vi "WebPowerSwitch.vi"() -> ()   [LabVIEW 2016]
uses:
  <vilib>/httpClient/LabVIEWHTTPClient.lvlib
panel:
  in  "url 2":string="http://LV:LV@192.168.126.155/outlet?a=OFF"
  out "error out":errorcluster
  out "body":string
  out "headers":string
  in  "url":string="http://LV:LV@192.168.126.155/index.htm"
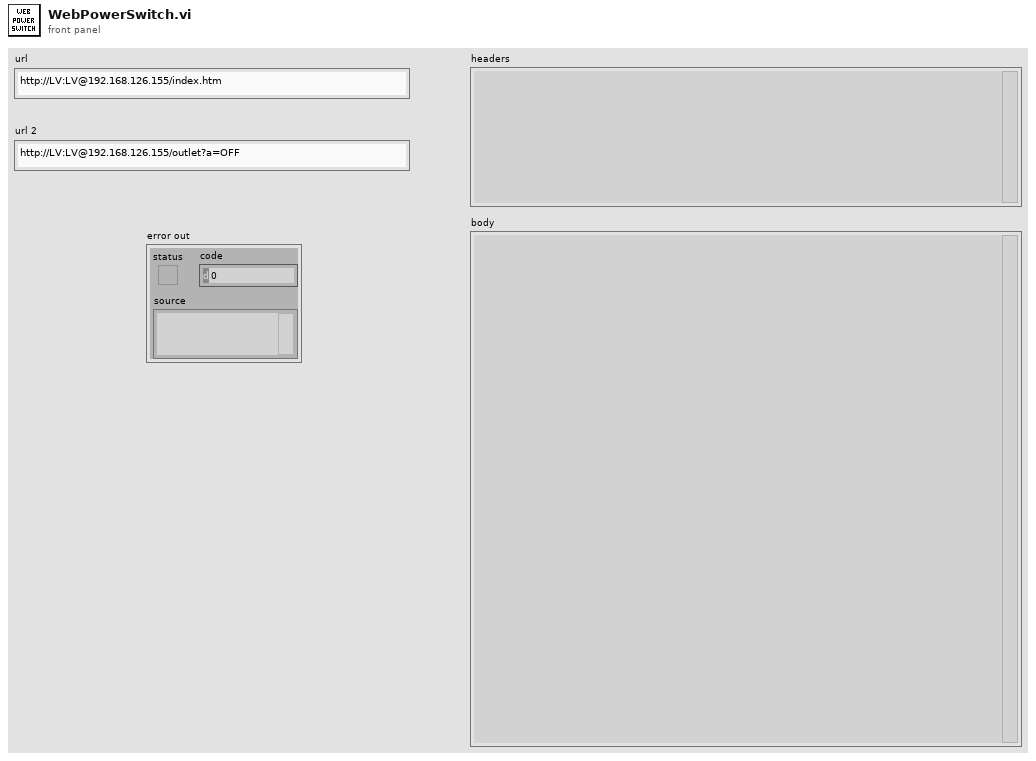
[diagram p1: front panel]
types:
  T1 = typedef "LabVIEWHTTPClient.lvlib/ClientHandle.ctl" = refnum<k1>
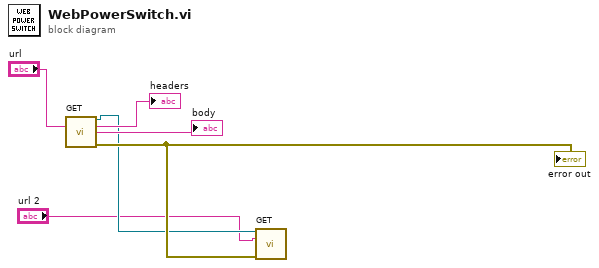
[diagram p0: block diagram]
diagram:
  n1 = call <vilib>:"GET.vi"("url"="url") -> ("client handle out"=w2:T1, "headers"=→"headers":string, "body"=→"body":string, "error out"=w3:errorcluster)  [unwired: 11 in]
  "error out" <- w3
  n2 = call <vilib>:"GET.vi"("client handle"=w2, "url"="url 2", "error in (no error)"=w3) -> ()  [unwired: 9 in, 4 out]
